vi "Create Serial Slave.vi"(4 "flow control":u16(ring) items=["None", "XON/XOFF", "RTS/CTS", "XON/XOFF & RTS/CTS", "DTR/DSR", "XON/XOFF & DTR/DSR"], 5 "serial type":enum16{"RTU", "ASCII"}(ring), 6 "parity (even)":u16(ring)=2 items=["None", "Odd", "Even", "Mark", "Space"], 7 "unit ID":u8=1, 8 "error in":errorcluster, 9 "device data model":refnum<class "Device Data Model.lvclass">, 10 "baud rate (9600)":u32=9600, 11 "VISA resource name":refnum<visa-resource-name>) -> (0 "error out":errorcluster, 3 "serial slave instance":refnum<class "Modbus Slave.lvclass">)   [LabVIEW 2021, in "API Main.lvlib"]
doc: "Creates a standard TCP slave with an IP ADU. If the data model input is unwired, a standard data model will be initialized and used. If the input is wired, the code will check to make sure that it is not the default value for the class (it should be initialized). If the default value of the class is wired, the standard model will be initialized and used."
uses:
  API Main.lvlib
  Slave/Modbus Slave.lvclass
  Data Model/Device Data Model.lvclass
  Transmission Data Unit/RTU/RTU Data Unit.lvclass
  D:/my_projects/projects/Algorithms/Labview/21/Modbus_v121c/Transmission Data Unit/Serial Interface/Serial Data Unit.lvclass
  Transmission Data Unit/ASCII/ASCII Data Unit.lvclass
  Transmission Data Unit/Transmission Data Unit.lvclass/Transmission Data Unit.ctl
  Network Protocol/Network Slave/Serial/Serial Slave.lvclass
  D:/my_projects/projects/Algorithms/Labview/21/Modbus_v121c/Network Protocol/Network Slave/Network Slave.lvclass
  Data Model/Standard Data Model/Standard Data Model.lvclass
  D:/my_projects/projects/Algorithms/Labview/21/Modbus_v121c/Data Model/Device Data Model.lvclass
  Transmission Data Unit/Serial Interface/Serial Data Unit.lvclass/Serial Data Unit.ctl
  Network Protocol/Network Slave/Network Slave.lvclass/Network Slave.ctl
  Slave/Modbus Slave.lvclass/Modbus Slave.ctl
  Data Model/Device Data Model.lvclass/Device Data Model.ctl
  Transmission Data Unit/Serial Interface/Write baud rate.vi
  Transmission Data Unit/Serial Interface/Write flow control.vi
  Transmission Data Unit/Serial Interface/Write parity.vi
  Transmission Data Unit/Serial Interface/Write visa resource name.vi
  Data Model/Read Initialized.vi
  <vilib>/Utility/error.llb/Clear Errors.vi
  Transmission Data Unit/Serial Interface/Serial Data Unit.lvclass
  D:/my_projects/projects/Algorithms/Labview/21/Modbus_v121c/Transmission Data Unit/Transmission Data Unit.lvclass
  Transmission Data Unit/Transmission Data Unit.lvclass
  Network Protocol/Network Slave/Network Slave.lvclass
panel:
  # "disable parity disallowed by mbspec"
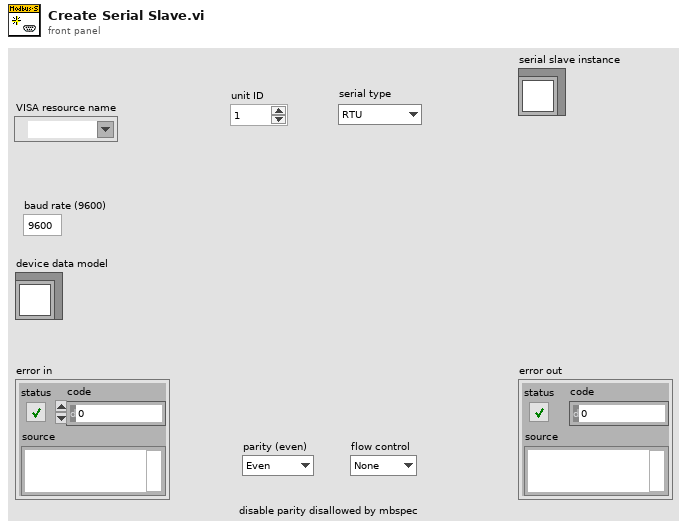
[diagram p1: front panel]
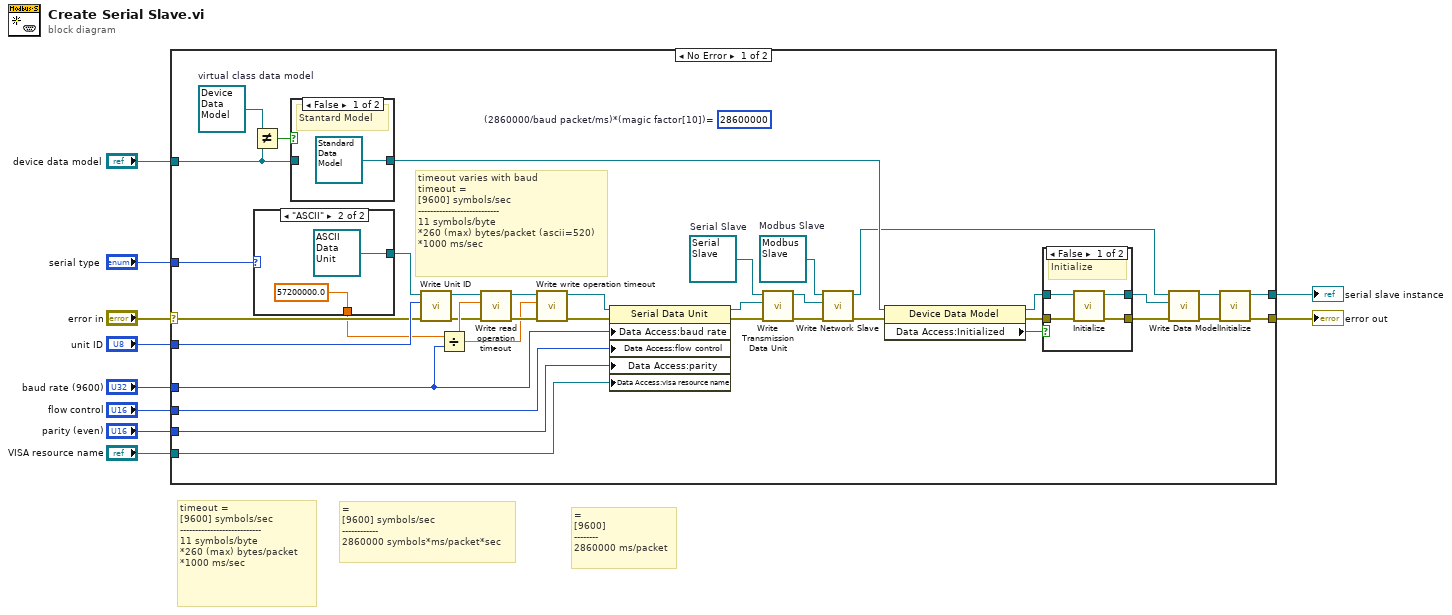
[diagram p0: block diagram]
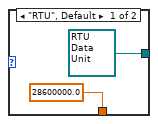
[diagram p3: hidden frame]
diagram:
  # "=\n[9600]\n--------\n2860000 ms/packet"
  # "=\n[9600] symbols/sec\n------------\n2860000 symbols*ms/packet*sec"
  # "timeout =\n[9600] symbols/sec\n---------------------------\n11 symbols/byte\n*260 (max) bytes/packet\n*1000 ms/sec"
  n1 = case shown="No Error" "error in" {
    selector: "error in" -> [w31 w60]
    tunnel: "VISA resource name" -> [w47 _]
    tunnel: [w46 w60] -> w4
    tunnel: "baud rate (9600)" -> [w23 _]
    tunnel: "flow control" -> [w45 _]
    tunnel: "parity (even)" -> [w44 _]
    tunnel: "serial type" -> [w43 _]
    tunnel: "device data model" -> [w37 _]
    tunnel: "unit ID" -> [w33 _]
    tunnel: [w32 _] -> w5
    frame No Error {
      w21 = refnum<class "Serial Slave.lvclass"> refnum  # Serial Slave
      (unwired) u32 28600000  # (2860000/baud packet/ms)*(magic factor[10])=
      w39 = refnum<class "Device Data Model.lvclass"> refnum  # virtual class data model
      w18 = refnum<class "Modbus Slave.lvclass"> refnum  # Modbus Slave
      # "timeout varies with baud\ntimeout =\n[9600] symbols/sec\n---------------------------\n11 symbols/byte\n*260 (max) bytes/packet (ascii=520)\n*1000 ms/sec"
      n2 = Not Equal?(x=w39, y=w37) -> (x != y?=w38:bool)
      n3 = case shown="\"ASCII\"" w43 {
        tunnel: [refnum<class "RTU Data Unit.lvclass"> refnum ("RTU Data Unit") refnum<class "ASCII Data Unit.lvclass"> refnum ("ASCII Data Unit")] -> w34
        tunnel: [28600000.0 ("x") 57200000.0 ("x")] -> w25
        frame "RTU", Default {
        }
        frame "ASCII" {
        }
      }
      n4 = case shown="False" w38 {
        tunnel: w37 -> [_ w49]
        tunnel: [refnum<class "Standard Data Model.lvclass"> refnum ("Standard Data Model") w49] -> w36
        frame False {
          # "Stantard Model"
        }
        frame True {
        }
      }
      n5 = call "Write Unit ID.vi"("error in"=w31, "unit ID"=w33, "transmission data unit in"=w34) -> ("error out"=w26:errorcluster, "transmission data unit out"=w27:refnum<class "Serial Data Unit.lvclass">)  [unwired: 7 in]
      n6 = Divide(x=w25, y=w23) -> (x/y=w28:dbl)
      n7 = call "Write read operation timeout.vi"("error in (no error)"=w26, "read operation timeout"=w28, "transmission data unit in"=w27) -> ("error out"=w29:errorcluster, "transmission data unit out"=w30:refnum<class "Serial Data Unit.lvclass">)  [unwired: 7 in]
      n8 = call "Write write operation timeout.vi"("error in (no error)"=w29, "write operation timeout"=w28, "transmission data unit in"=w30) -> ("error out"=w22:errorcluster, "transmission data unit out"=w13:refnum<class "Serial Data Unit.lvclass">)  [unwired: 7 in]
      n9 = property class="Serial Data Unit"(reference=w13, error in=w22, "Data Access:baud rate"=w23, "Data Access:flow control"=w45, "Data Access:parity"=w44, "Data Access:visa resource name"=w47) -> (reference out=w12:refnum<class "Serial Data Unit.lvclass">, error out=w11:errorcluster)
      n10 = call "Write Transmission Data Unit.vi"("error in (no error)"=w11, "Transmission Data Unit"=w12, "Network Slave in"=w21) -> ("error out"=w20:errorcluster, "Network Slave out"=w19:refnum<class "Serial Slave.lvclass">)  [unwired: 7 in]
      n11 = call "Write Network Slave.vi"("error in (no error)"=w20, "Network Slave"=w19, "Modbus Slave in"=w18) -> ("error out"=w17:errorcluster, "Modbus Slave out"=w16:refnum<class "Modbus Slave.lvclass">)  [unwired: 7 in]
      n12 = property class="Device Data Model"(reference=w36, error in=w17) -> (reference out=w41:refnum<class "Device Data Model.lvclass">, error out=w42:errorcluster, "Data Access:Initialized"=w40:bool)
      n13 = case shown="False" w40 {
        tunnel: w42 -> [w57 w59]
        tunnel: [w56 w59] -> w24
        tunnel: [w55 w58] -> w35
        tunnel: w41 -> [w54 w58]
        frame False {
          # "Initialize"
          n14 = call-dynamic "Initialize.vi"("error in"=w57, "device data model in"=w54) -> ("error out"=w56:errorcluster, "device data model out"=w55:refnum<class "Device Data Model.lvclass">)  [unwired: 8 in]
        }
        frame True {
        }
      }
      n15 = call "Write Data Model.vi"("error in (no error)"=w24, "device data model"=w35, "Modbus slave in"=w16) -> ("error out"=w14:errorcluster, "Modbus slave out"=w15:refnum<class "Modbus Slave.lvclass">)  [unwired: 7 in]
      n16 = call-dynamic "Initialize.vi"("error in (no error)"=w14, "Modbus slave in"=w15) -> ("error out"=w46:errorcluster, "Modbus slave out"=w32:refnum<class "Modbus Slave.lvclass">)  [unwired: 8 in]
    }
    frame Error {
    }
  }
  "error out" <- w4
  "serial slave instance" <- w5
